vi "Giffler Thompson Active Schedule Engine.vi"(8 "Number of  Jobs":i32=4, 9 "Number of Machines":i32=4, 10 "Processing Times":u16[][](array[numeric])=[[34, 15, 38, 95], [2, 89, 19, 7], [54, 70, 28, 34], [61, 9, 87, 29]], 11 "Schedule In":u16[](array[numeric])=[12, 0, 7, 2, 6, 3, 13, 5, 1, 4, 14, 11, 10, 15, 8, 9]) -> (0 "Machine Completion Times":u16[](array[numeric]), 1 "Job Completion Times":u16[](array[numeric]), 2 "Completion Times":u16[][](array[numeric]), 3 "Start Times":u16[][](array[numeric]), 4 "Schedule Order":u16[](array[numeric]))   [LabVIEW 2013, in "GanntChart.lvclass"]
uses:
  GanntChart.lvclass
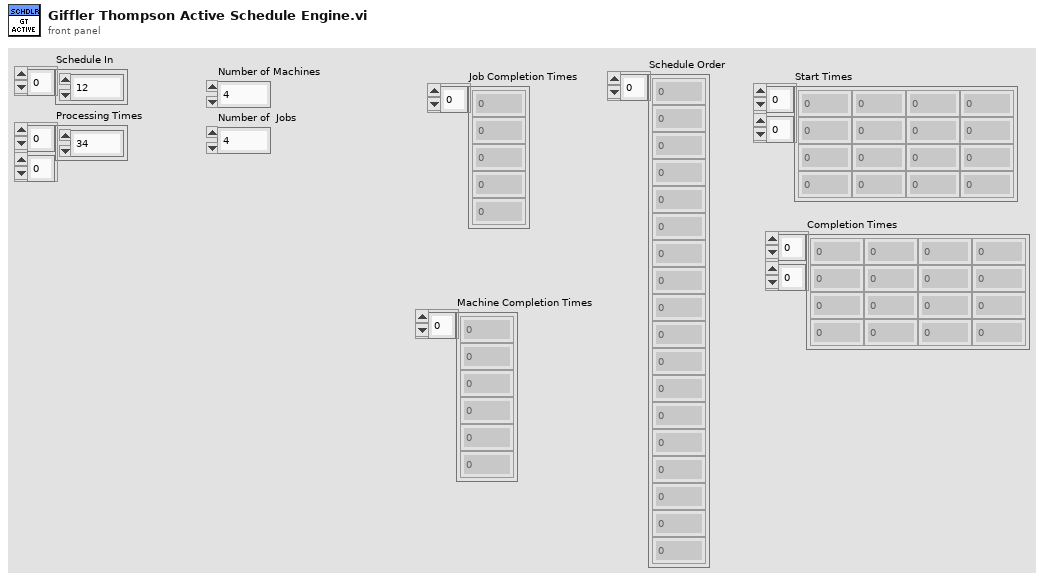
[diagram p1: front panel]
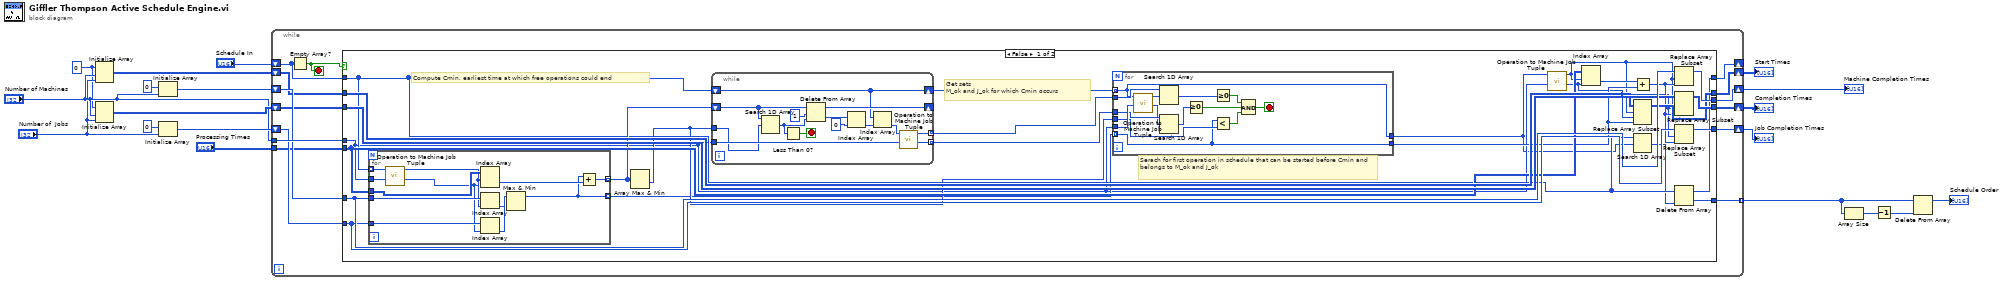
[diagram p0: block diagram]
diagram:
  w7 = u16 0 ("element")
  n1 = Initialize Array(w7, "Number of Machines", "Number of  Jobs") -> (w6:u16[][])
  n2 = Initialize Array(w7, "Number of Machines", "Number of  Jobs") -> (w14:u16[][])
  n3 = Initialize Array(u16 0 ("element"), "Number of Machines") -> (w16:u16[])
  n4 = Initialize Array(u16 0 ("element"), "Number of  Jobs") -> (w17:u16[])
  n5 = while {
    shift-right: [w25] -> _
    shift-left: "Schedule In" -> [w32]
    tunnel: "Number of Machines" -> [w31]
    shift-right: [w28] -> w12
    shift-left: w17 -> [w30]
    shift-right: [w27] -> w11
    shift-left: w16 -> [w29]
    shift-right: [w23] -> w13
    shift-left: w14 -> [w24]
    tunnel: "Processing Times" -> [w26]
    shift-right: [w21] -> w5
    shift-left: w6 -> [w22]
    tunnel: [w20] -> w1 mode=indexing
    stop <- w33 stop-if-true
    n6 = Empty Array?(array=w32) -> (empty?=w33:bool)
    n7 = case shown="False" w33 {
      tunnel: w32 -> [w48 w102]
      tunnel: w31 -> [w42 _]
      tunnel: w30 -> [w58 w104]
      tunnel: w29 -> [w59 w103]
      tunnel: [w57 w104] -> w28
      tunnel: [w56 w103] -> w27
      tunnel: w26 -> [w51 _]
      tunnel: [w35 w102] -> w25
      tunnel: w24 -> [w55 w101]
      tunnel: [w54 w101] -> w23
      tunnel: w22 -> [w53 w100]
      tunnel: [w52 w100] -> w21
      tunnel: [w34 _] -> w20
      frame False {
        # "Serach for first operation in schedule that can be started before Cmin and belongs to M_ok and J_ok"
        # "Get sets \nM_ok and J_ok for which Cmin occurs"
        # "Compute Cmin, earliest time at which free operations could end"
        n8 = for {
          tunnel: w48 -> [w99] mode=indexing
          tunnel: w42 -> [w98]
          tunnel: w58 -> [w96]
          tunnel: w59 -> [w97]
          tunnel: [w89] -> w49 mode=indexing
          tunnel: w51 -> [w93]
          tunnel: [w88] -> w44 mode=indexing
          n9 = call "Operation to Machine Job Tuple.vi"("Number of Machines"=w98, "Operation Number"=w99) -> ("Job No"=w91:i32, "Machine No"=w92:i32)  [unwired: 8 in]
          n10 = Index Array(array=w93, index (row)=w92, index (col)=w91) -> (element=w90:u16)
          n11 = Index Array(array=w97, index=w92) -> (element=w94:u16)
          n12 = Index Array(array=w96, index=w91) -> (element=w95:u16)
          n13 = Max & Min(x=w95, y=w94) -> (max(x,y)=w88:u16)  [unwired: 1 out]
          n14 = Add(x=w88, y=w90) -> (x+y=w89:u16)
        }
        n15 = Array Max & Min(array=w49) -> (min value=w47:u16)  [unwired: 3 out]
        n16 = while {
          shift-right: [w83] -> _
          shift-left: w49 -> [w85]
          tunnel: w47 -> [w75]
          tunnel: w42 -> [w78]
          tunnel: [w77] -> w46 mode=indexing
          tunnel: [w76] -> w45 mode=indexing
          shift-right: [w74] -> w43
          shift-left: w48 -> [w74]
          stop <- w87 stop-if-true
          n17 = Search 1D Array(1D array=w85, element=w75) -> (index of element=w86:i32)  [unwired: 1 in]
          n18 = Less Than 0?(x=w86) -> (x < 0?=w87:bool)
          n19 = Delete From Array(array=w85, length=1, index=w86) -> (deleted portion=w82:u16[], array with subset deleted=w83:u16[])
          n20 = Index Array(array=w82, index=0) -> (element=w80:u16)
          n21 = Index Array(array=w74, index=w80) -> (element=w79:u16)
          n22 = call "Operation to Machine Job Tuple.vi"("Number of Machines"=w78, "Operation Number"=w79) -> ("Job No"=w76:i32, "Machine No"=w77:i32)  [unwired: 8 in]
        }
        n23 = for {
          tunnel: w43 -> [w60] mode=indexing
          tunnel: w42 -> [w73]
          tunnel: w44 -> [w61] mode=indexing
          tunnel: w46 -> [w72]
          tunnel: w45 -> [w69]
          tunnel: w47 -> [w66]
          tunnel: [w61] -> w50
          tunnel: [w60] -> w37
          stop <- w62 stop-if-true
          n24 = call "Operation to Machine Job Tuple.vi"("Number of Machines"=w73, "Operation Number"=w60) -> ("Job No"=w68:i32, "Machine No"=w71:i32)  [unwired: 8 in]
          n25 = Search 1D Array(1D array=w72, element=w71) -> (index of element=w70:i32)  [unwired: 1 in]
          n26 = Search 1D Array(1D array=w69, element=w68) -> (index of element=w67:i32)  [unwired: 1 in]
          n27 = Greater Or Equal To 0?(x=w67) -> (x >= 0?=w64:bool)
          n28 = Less?(x=w61, y=w66) -> (x < y?=w63:bool)
          n29 = Greater Or Equal To 0?(x=w70) -> (x >= 0?=w65:bool)
          n30 = Compound Arithmetic op=AND(w65, w64, w63) -> (w62:bool)
        }
        n31 = call "Operation to Machine Job Tuple.vi"("Number of Machines"=w42, "Operation Number"=w37) -> ("Job No"=w38:i32, "Machine No"=w39:i32)  [unwired: 8 in]
        n32 = Index Array(array=w51, index (row)=w39, index (col)=w38) -> (element=w41:u16)
        n33 = Replace Array Subset(array=w53, new element=w50, index (row)=w39, index (col)=w38) -> (w52:u16[][])
        n34 = Search 1D Array(1D array=w48, element=w37) -> (index of element=w36:i32)  [unwired: 1 in]
        n35 = Add(x=w41, y=w50) -> (x+y=w40:u16)
        n36 = Replace Array Subset(array=w59, new element=w40, index=w39) -> (w56:u16[])
        n37 = Replace Array Subset(array=w55, new element=w40, index (row)=w39, index (col)=w38) -> (w54:u16[][])
        n38 = Replace Array Subset(array=w58, new element=w40, index=w38) -> (w57:u16[])
        n39 = Delete From Array(array=w48, index=w36) -> (deleted portion=w34:u16, array with subset deleted=w35:u16[])  [unwired: 1 in]
      }
      frame True {
      }
    }
  }
  "Completion Times" <- w13
  "Job Completion Times" <- w12
  "Machine Completion Times" <- w11
  "Start Times" <- w5
  n40 = Array Size(array=w1) -> (size(s)=w4:i32)
  n41 = Decrement(x=w4) -> (x-1=w3:i32)
  n42 = Delete From Array(array=w1, index=w3) -> (array with subset deleted=→"Schedule Order":u16[])  [unwired: 1 in, 1 out]
